vi "geve-timer_loop.vi"() -> (3 "loop time (ms)":u32)   [LabVIEW 2018]
doc: "simple timer loop vi used for debugging if needed"
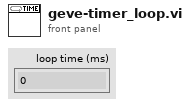
[diagram p1: front panel]
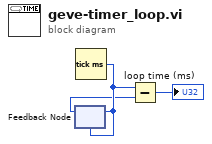
[diagram p0: block diagram]
diagram:
  n1 = Tick Count (ms)() -> (millisecond timer value=w3:u32)
  n2 = feedback #1(w3) -> (w1:u32)
  n3 = feedback-in #1(w3) -> ()
  n4 = Subtract(x=w3, y=w1) -> (x-y=→"loop time (ms)":u32)
